vi "demo.vi"() -> ()   [LabVIEW 2015]
uses:
  dll/cbLib.dll
  dll/LvWrap.dll
panel:
  out "Int32Val":i32
  out "EventRef_i32val":u32 format="%08x"
  out "Time":string
  out "Waveform Chart":u32(graph)
  in  "interval_ms":u32=100 format="%d ms"
  in  "btn_Stop":bool
  in  "btn_Start":bool
  out "randomNum":u32
  out "EventRef_u8arr":u32 format="%08x"
  out "errCode":i32
  out "CallBackFunc Handle":u32 format="%08x"
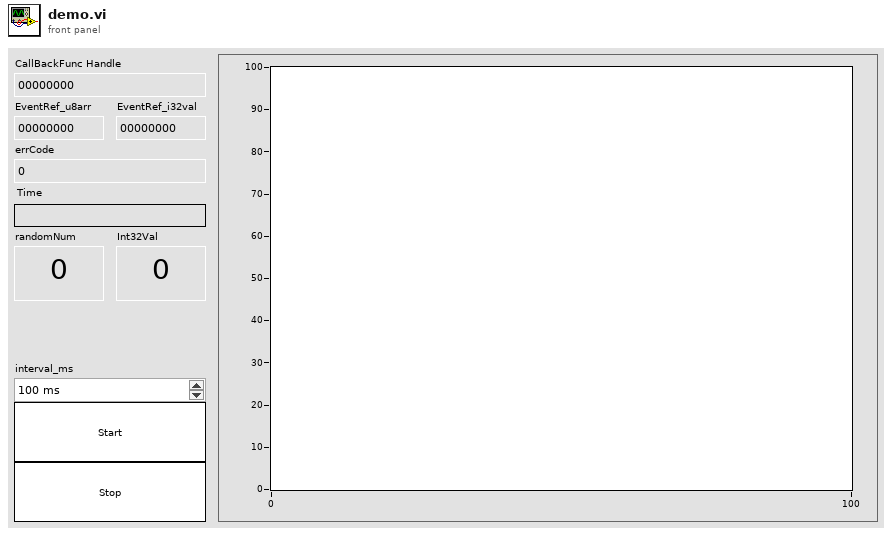
[diagram p1: front panel]
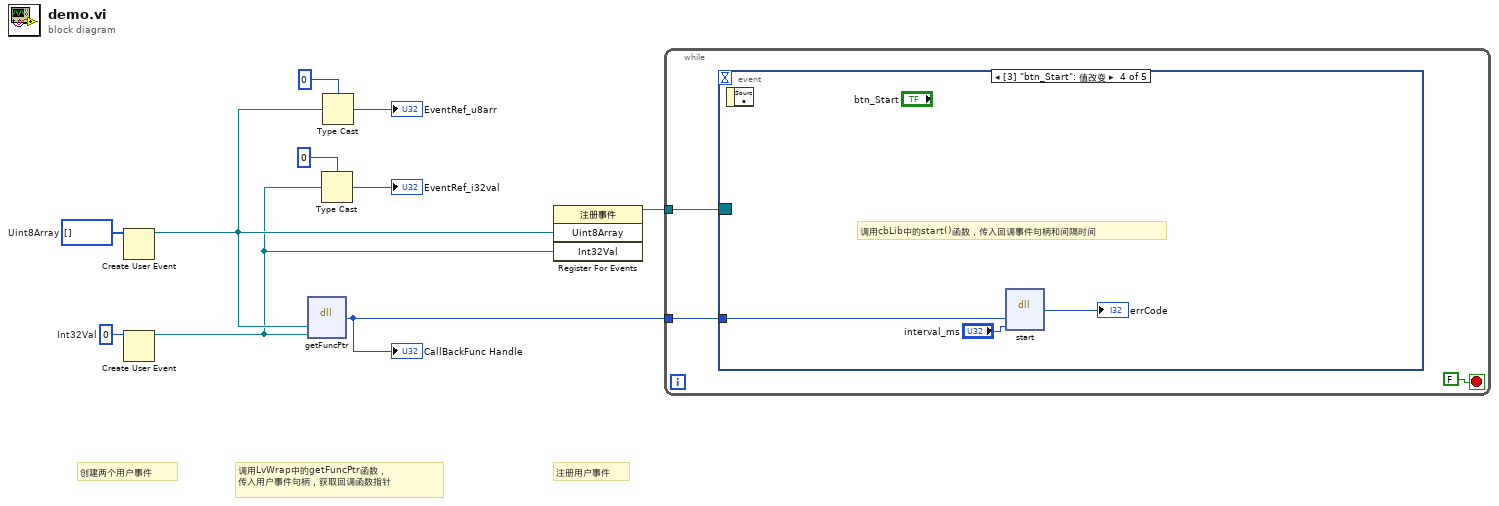
[diagram p0: block diagram]
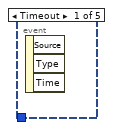
[diagram p2: hidden frame]
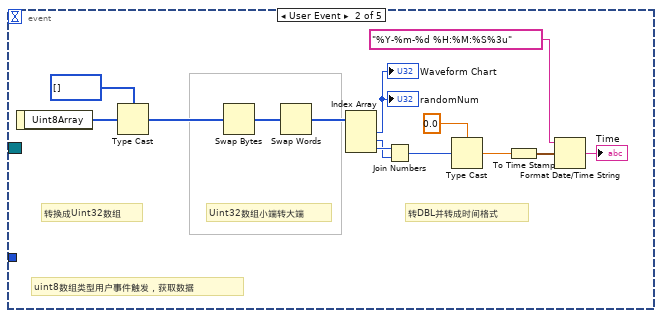
[diagram p3: hidden frame]
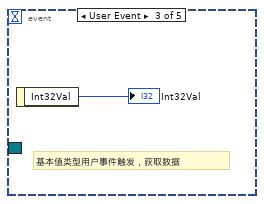
[diagram p4: hidden frame]
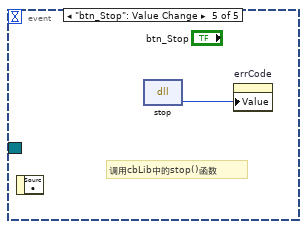
[diagram p5: hidden frame]
diagram:
  w4 = 0  # Int32Val
  w10 = u8[] []  # Uint8Array
  # "注册用户事件"
  # "调用LvWrap中的getFuncPtr函数，\n传入用户事件句柄，获取回调函数指针"
  # "创建两个用户事件"
  n1 = Create User Event(user event datatype=w10) -> (user event=w5:refnum<user-event>)  [unwired: 1 in, 1 out]
  n2 = Create User Event(user event datatype=w4) -> (user event=w1:refnum<user-event>)  [unwired: 1 in, 1 out]
  n3 = dll-call lib="D:/MyProjects/CLAN Studio Toolkits/Tutorial/LabVIEW DLL Callback/03-LvDemo/source/dll/LvWrap.dll" fn="getFuncPtr"("eventRef_uint8arr"=w5, "eventRef_int32val"=w1) -> ("cbFunc"=w8:u64)  [unwired: 5 in, 2 out]
  "CallBackFunc Handle" <- w8
  n4 = Type Cast(type=u32 0, x=w1) -> (*(type *) &x=→"EventRef_i32val":u32)
  n5 = Type Cast(type=u32 0, x=w5) -> (*(type *) &x=→"EventRef_u8arr":u32)
  n6 = register-events(w5, w1) -> (reference out=w9:refnum<event-registration>)  [unwired: 2 in, 1 out]
  n7 = while {
    tunnel: w9 -> [w12]
    tunnel: w8 -> [w11]
    stop <- FALSE stop-if-true
    n8 = event shown="[3] \"btn_Start\": 值改变" {
      selector: w12 -> [_ _ _ _ _]
      dyn-events: _ -> [_ _ _ _ _]
      timeout: _ -> [_ _ _ _ _]
      tunnel: w11 -> [_ _ _ w31 _]
      event Timeout {
        n9 = event-data() -> ()  [unwired: 1 in, 3 out]
      }
      event User Event {
        # "转DBL并转成时间格式"
        # "Uint32数组小端转大端"
        # "转换成Uint32数组"
        # "uint8数组类型用户事件触发，获取数据"
        n10 = event-data() -> ("Uint8Array"=w27:u8[])  [unwired: 1 in]
        n11 = Type Cast(type=u32[] [], x=w27) -> (*(type *) &x=w25:u32[])
        n12 = Swap Bytes(anything=w25) -> (byte swapped=w24:u32[])
        n13 = Swap Words(1:w24) -> (0:w23:u32[])
        n14 = Index Array(array=w23) -> (element #1=→"randomNum" →"Waveform Chart":u32, element #2=w21:u32, element #3=w22:u32)  [unwired: 3 in]
        n15 = Join Numbers(hi=w22, lo=w21) -> ((hi.lo)=w20:u64)
        n16 = Type Cast(type=0.0 ("数值"), x=w20) -> (*(type *) &x=w18:dbl)
        n17 = To Time Stamp(1:w18) -> (0:w15:timestamp)
        n18 = Format Date/Time String(time format string (%c)="%Y-%m-%d %H:%M:%S%3u" ("时间格式字符串(%c)"), seconds (now)=w15) -> (date/time string=→"Time":string)  [unwired: 1 in]
      }
      event User Event {
        # "基本值类型用户事件触发，获取数据"
        n19 = event-data() -> ("Int32Val"=→"Int32Val":i32)  [unwired: 1 in]
      }
      event "btn_Start": Value Change {
        # "调用cbLib中的start()函数，传入回调事件句柄和间隔时间"
        n20 = event-data() -> ()  [unwired: 1 in, 1 out]
        n21 = dll-call lib="D:/MyProjects/CLAN Studio Toolkits/Tutorial/LabVIEW DLL Callback/03-LvDemo/source/dll/cbLib.dll" fn="start"("callback"=w31, "interval_ms"="interval_ms") -> ("errCode"=→"errCode":i32)  [unwired: 5 in, 2 out]
      }
      event "btn_Stop": Value Change {
        # "调用cbLib中的stop()函数"
        n22 = event-data() -> ()  [unwired: 1 in, 1 out]
        n23 = dll-call lib="D:/MyProjects/CLAN Studio Toolkits/Tutorial/LabVIEW DLL Callback/03-LvDemo/source/dll/cbLib.dll" fn="stop"() -> ("errCode"=w32:i32)  [unwired: 3 in, 2 out]
        n24 = property on="errCode" class="DigNum (严格)"("Value"=w32) -> ()  [unwired: 2 in, 2 out]
      }
    }
  }
